vi "ftspike.vi"(6 "angle":dbl, 8 "size window":dbl, 9 "q3":dbl, 10 "q1":dbl, 11 "I":dbl[][](array[numeric])) -> (3 "output":dbl)   [LabVIEW 2020]
panel:
  out "contrast":dbl
  out "spike1":dbl
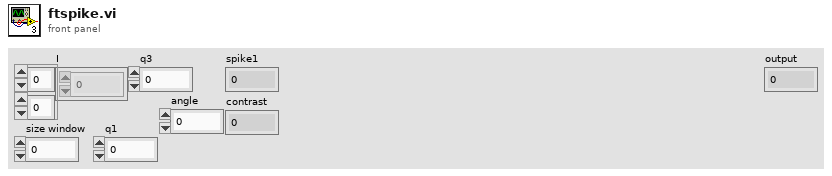
[diagram p1: front panel]
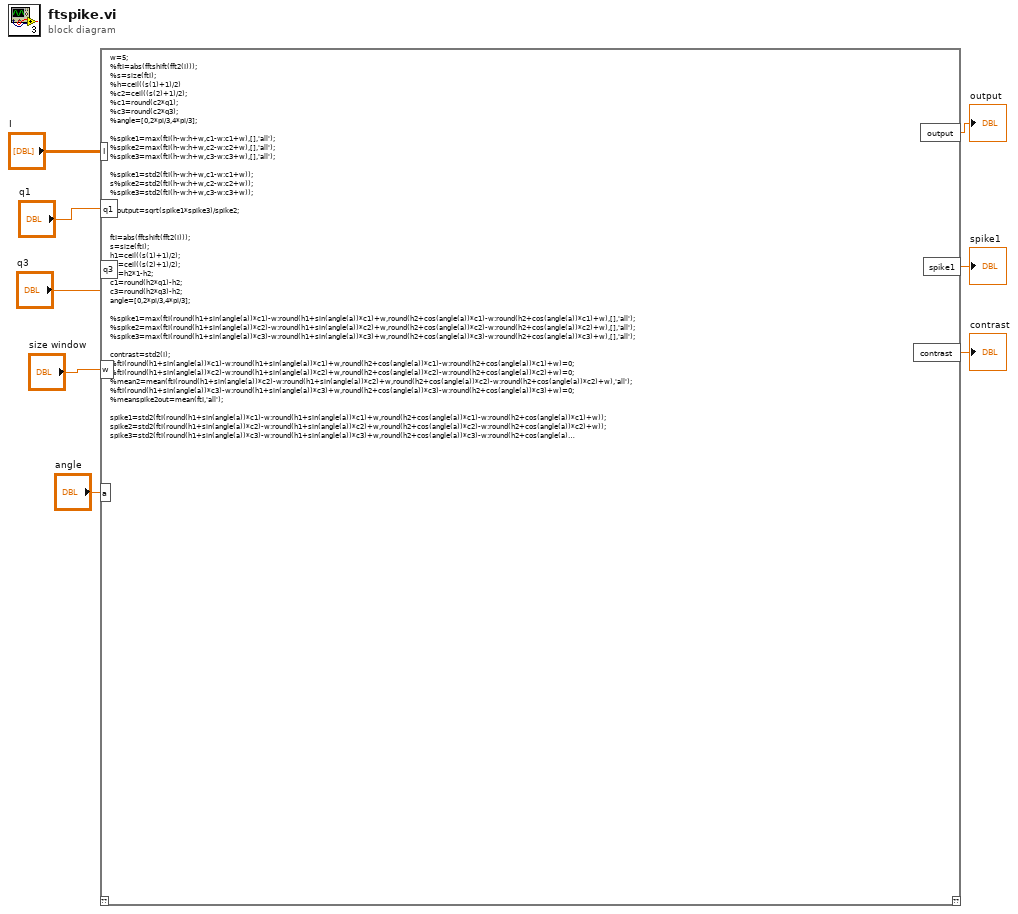
[diagram p0: block diagram]
diagram:
  n1 = script code="w=5;\n%ftI=abs(fftshift(fft2(I)));\n%s=size(ftI);\n%h=ceil((s(1)+1)/2)\n%c2=ceil((s(2)+1)/2);\n%c1=round(c2*q1);\n%c3=round(c2*q3);\n%angle=[0,2*pi/3,4*pi/3];\n\n%spike1=max(ftI(h-w:h+w,c1-w:c1+w),[],'all');\n%spike2=max(ftI(h-w:h+w,c2-w:c2+w),[],'all');\n%spike3=max(ftI(h-w:h+w,c3-w:c3+w),[],'all');\n\n%spike1=std2(ftI(h-w:h+w,c1-w:c1+w));\ns%pike2=std2(ftI(h-w:h+w,c2-w:c2+w));\n%spike3=std2(ftI(h-w:h+w,c3-w:c3+w));\n\n%output=sqrt(spike1*spike3)/spike2;\n\n\nftI=abs(fftshift(fft2(I)));\ns=size(ftI);\nh1=ceil((s(1)+1)/2);\nh2=ceil((s(2)+1)/2);\nc2=h2*1-h2;\nc1=round(h2*q1)-h2;\nc3=round(h2*q3)-h2;\nangle=[0,2*pi/3,4*pi/3];\n\n%spike1=max(ftI(round(h1+sin(angle(a))*c1)-w:round(h1+sin(angle(a))*c1)+w,round(h2+cos(angle(a))*c1)-w:round(h2+cos(angle(a))*c1)+w),[],'all');\n%spike2=max(ftI(round(h1+sin(angle(a))*c2)-w:round(h1+sin(angle(a))*c2)+w,round(h2+cos(angle(a))*c2)-w:round(h2+cos(angle(a))*c2)+w),[],'all');\n%spike3=max(ftI(round(h1+sin(angle(a))*c3)-w:round(h1+sin(angle(a))*c3)+w,round(h2+cos(angle(a))*c3)-w:round(h2+cos(angle(a))*c3)+w),[],'all');\n\ncontrast=std2(I);\n%ftI(round(h1+sin(angle(a))*c1)-w:round(h1+sin(angle(a))*c1)+w,round(h2+cos(angle(a))*c1)-w:round(h2+cos(angle(a))*c1)+w)=0;\n%ftI(round(h1+sin(angle(a))*c2)-w:round(h1+sin(angle(a))*c2)+w,round(h2+cos(angle(a))*c2)-w:round(h2+cos(angle(a))*c2)+w)=0;\n%mean2=mean(ftI(round(h1+sin(angle(a))*c2)-w:round(h1+sin(angle(a))*c2)+w,round(h2+cos(angle(a))*c2)-w:round(h2+cos(angle(a))*c2)+w),'all');\n%ftI(round(h1+sin(angle(a))*c3)-w:round(h1+sin(angle(a))*c3)+w,round(h2+cos(angle(a))*c3)-w:round(h2+cos(angle(a))*c3)+w)=0;\n%meanspike2out=mean(ftI,'all');\n\nspike1=std2(ftI(round(h1+sin(angle(a))*c1)-w:round(h1+sin(angle(a))*c1)+w,round(h2+cos(angle(a))*c1)-w:round(h2+cos(angle(a))*c1)+w));\nspike2=std2(ftI(round(h1+sin(angle(a))*c2)-w:round(h1+sin(angle(a))*c2)+w,round(h2+cos(angle(a))*c2)-w:round(h2+cos(angle(a))*c2)+w));\nspike3=std2(ftI(round(h1+sin(angle(a))*c3)-w:round(h1+sin(angle(a))*c3)+w,round(h2+cos(angle(a))*c3)-w:round(h2+cos(angle(a))*c3)+w));\n\noutput=sqrt(spike1*spike3)/spike2;\n%output=sqrt(spike1*spike3);\n%output=sqrt(spike1*spike3)/contrast;\n%output=sqrt(spike1*spike3)/mean(ftI,'all');\n%output=sqrt(spike1*spike3)/mean2;\n%output=spike1*spike3/contrast;\n%output=spike1*spike3/meanspike2out;\n%output=contrast;"("I"="I", "w"="size window", "q1"="q1", "q3"="q3", "a"="angle") -> ("output"=→"output":dbl, "spike1"=→"spike1":dbl, "contrast"=→"contrast":dbl)  [unwired: 1 in, 1 out]
